vi "IFwTemplate.vi"() -> ()   [LabVIEW 2015]
uses:
  <vilib>/Platform/TimedLoop/XDataNode/timing_clust.ctl
  <vilib>/Platform/TimedLoop/XDataNode/nitl_modes.ctl
  <vilib>/Platform/TimedLoop/XDataNode/wakeup.ctl
  <vilib>/rvi/Emulation/niFpgaGetClockAttributes.vi
  <vilib>/rvi/Emulation/niFpgaSctlEmulationGetInTimedLoop.vi
  <vilib>/rvi/Emulation/niFpgaEmulationReportErrorSimple.vi
  <vilib>/rvi/Emulation/niFpgaCriticalErrorInLSC.vi
  <vilib>/Platform/TimedLoop/XDataNode/XDataNode.xnode
  <instrlib>/_niInstr/FIFO Register Bus/v1/FPGA/niInstr FIFO Register Bus v1 FPGA.lvclass
  <vilib>/Platform/TimedLoop/XDataNode/XDNodeRunTimeDep.lvlib
  <instrlib>/_niInstr/Instruction Framework/v1/FPGA/Top Level Bus/Register Configuration/Register Configuration.lvclass
  IFw_Addon/FPGA/WaveformAddressSpace.lvclass
panel:
  in  "injectError0":errorcluster
  in  "fifo reg bus ctrl 0":u32
  out "fifo reg bus status 0":u32
  out "fifo reg bus data 0":u64
  # "Total Slices: 32.8% (4357 out of 13300)\nSlice Registers: 11.5% (12270 out of 106400)\nSlice LUTs: 21.7% (11527 out of 53200)\nBlock RAMs: 6.4% (9 out of 140)\nDSP48s: 0.0% (0 out of 220)"
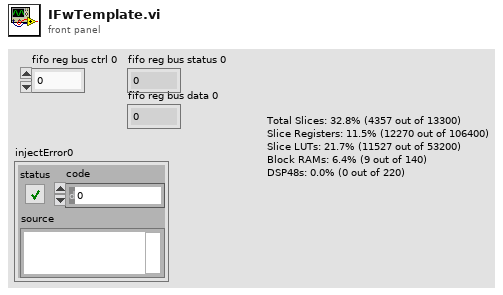
[diagram p1: front panel]
types:
  T1 = typedef "XDNodeRunTimeDep.lvlib/timing_clust.ctl" = cluster{"Expected End [f-1]":u64, "Actual End [f-1]":u64, "Finished Late? [f-1]":bool, "Expected End [i-1]":u64, "Actual End [i-1]":u64, "Finished Late? [i-1]":bool, "Expected Start [i]":u64, "Actual Start [i]":u64, "Expected Start [f]":u64, "Actual Start [f]":u64, "Source Name":string, "Structure Name":string, "Period":i64, "Deadline":i64, "Offset":i64, "Start":i64, "Priority":i32, "Timeout":i32, "Mode":T2, "Wakeup Reason":T3, "Error":errorcluster, "Source Type":string, "Secondary Source Type":string, "Global End Time":u64, "Global Start Time":u64, "Frame Duration":u64, "Iteration Duration":u64, "Assigned CPU":i32, "I/O Scan Engine Mode":u32}
  T2 = typedef "XDNodeRunTimeDep.lvlib/nitl_modes.ctl" = enum32{"No Change", "Process missed periods, maintain original phase", "Discard missed periods, maintain original phase", "Process missed periods, ignore original phase", "Discard missed periods, ignore original phase"}
  T3 = typedef "XDNodeRunTimeDep.lvlib/wakeup.ctl" = enum32{"Normal", "Aborted", "Asynchronous wakeup", "Timing source error", "Timed loop error", "Timeout"}
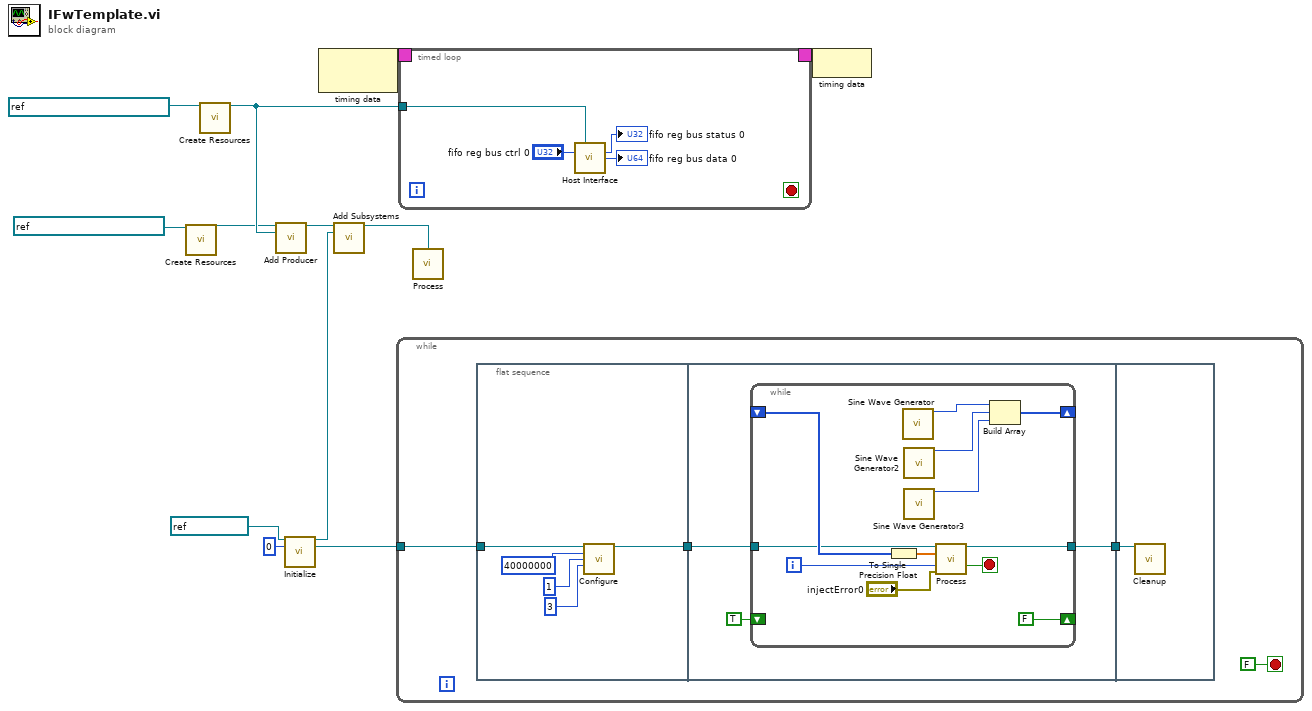
[diagram p0: block diagram]
diagram:
  n1 = call <instrlib>:"Create Resources.vi"("register clock"=refnum<k21> "40 MHz Onboard Clock") -> ("register configuration"=w8:refnum<class "Register Configuration.lvclass">)  [unwired: 14 in]
  n2 = call <instrlib>:"Create Resources.vi"("instruction fifo"=refnum<k21> "reg.host instruction fifo 0") -> ("fifo register bus"=w9:refnum<class "niInstr FIFO Register Bus v1 FPGA.lvclass">)  [unwired: 14 in]
  n3 = call <instrlib>:"Add Producer.vi"("register configuration in"=w8, "instruction producer"=w9) -> ("register configuration out"=w6:refnum<class "Register Configuration.lvclass">)  [unwired: 13 in]
  n4 = call "Initialize.vi"("DMA FIFO"=refnum<k21> "DataSGL0" ("FIFO Out"), "instance"=u8 0) -> ("subsystem"=w2:refnum<class "Single Address Space Collection.lvclass">, "AddressSpace"=w3:refnum<class "WaveformAddressSpace.lvclass">)  [unwired: 12 in]
  n5 = node-c288() -> (w12:T1)  [unwired: 1 in]
  n6 = call <instrlib>:"Add Subsystems.vi"("register configuration in"=w6, "subsystems"=w2) -> ("register configuration out"=w1:refnum<class "Register Configuration.lvclass">)  [unwired: 13 in]
  n7 = while {
    tunnel: w3 -> [w13]
    stop <- FALSE stop-if-true
    n8 = flat-sequence {
      tunnel: [w17] -> w15
      tunnel: w13 -> [w18]
      tunnel: w15 -> [w24]
      tunnel: [w23] -> w14
      tunnel: w14 -> [w37]
      frame #0 {
        n9 = call "Configure.vi"("WaveformAddressSpace in"=w18, "oclk_freq"=u32 40000000, "oclk_mult"=u32 1, "UnderflowMargin"=u32 3 ("y")) -> ("WaveformAddressSpace out"=w17:refnum<class "WaveformAddressSpace.lvclass">)  [unwired: 11 in]
      }
      frame #1 {
        n10 = while {
          shift-right: [w33] -> _
          shift-left: _ -> [w35]
          shift-right: [FALSE] -> _
          shift-left: TRUE -> [_]
          tunnel: w24 -> [w28]
          tunnel: [w27] -> w23
          i -> [w34]
          stop <- w30 stop-if-true
          n11 = To Single Precision Float(number=w35) -> (single precision float=w29:sgl[])
          n12 = call "Sine Wave Generator"() -> ("sine out"=w32:i16)  [unwired: 15 in]
          n13 = call "Sine Wave Generator2"() -> ("sine out"=w26:i16)  [unwired: 15 in]
          n14 = call "Sine Wave Generator3"() -> ("sine out"=w25:i16)  [unwired: 15 in]
          n15 = call <instrlib>:"Process.vi"("WaveformAddressSpace in"=w28, "Data"=w29, "Iteration"=w34, "error in (no error)"="injectError0") -> ("WaveformAddressSpace out"=w27:refnum<class "WaveformAddressSpace.lvclass">, "stop"=w30:bool)  [unwired: 8 in, 2 out]
          n16 = Build Array(w32, w26, w25) -> (w33:i16[])
        }
      }
      frame #2 {
        n17 = call "Cleanup.vi"("WaveformAddressSpace in"=w37) -> ()  [unwired: 14 in, 1 out]
      }
    }
  }
  n18 = timed-loop {
    timing: w12 -> [_]
    timing-out: [_] -> w11
    tunnel: w9 -> [w41]
    stop <- _ stop-if-true
    n19 = call <instrlib>:"Host Interface.vi"("fifo register bus"=w41, "fifo reg bus ctrl 0"="fifo reg bus ctrl 0") -> ("fifo reg bus status 0"=→"fifo reg bus status 0":u32, "fifo reg bus data 0"=→"fifo reg bus data 0":u64)  [unwired: 12 in]
  }
  n20 = call <instrlib>:"Process.vi"("register configuration"=w1) -> ()  [unwired: 15 in]
  n21 = node-c288(w11) -> ()
